vi "random phase generator.vi"(0 "seed":u32=4294967295, 1 "reset":bool) -> (4 "white noise out":i16)   [LabVIEW 2012]
doc: "Generates a white noise signal with uniform or Gaussian distribution.\n--------------------\n\nThis Express VI is configured as follows:\n\n<b>White Noise Type</b>\nUniform\n\n<b>Execution Mode</b>\nOutside single-cycle Timed Loop\n\n<b>Scaling</b>\nAmplitude: 256 \n\n<b>Output Data Type</b>\nI16"
uses:
  <vilib>/Platform/TimedLoop/XDataNode/timing_clust.ctl
  <vilib>/Platform/TimedLoop/XDataNode/nitl_modes.ctl
  <vilib>/Platform/TimedLoop/XDataNode/wakeup.ctl
  <vilib>/rvi/Emulation/niFpgaSctlEmulationRegisterWithScheduler.vi
  <vilib>/rvi/Emulation/niFpgaSctlEmulationScheduler.vi
  <vilib>/Platform/TimedLoop/XDataNode/XDataNode.xnode
  <vilib>/Platform/TimedLoop/XDataNode/XDNodeRunTimeDep.lvlib
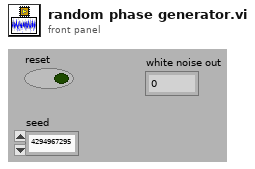
[diagram p1: front panel]
types:
  T1 = typedef "XDNodeRunTimeDep.lvlib/timing_clust.ctl" = cluster{"Expected End [f-1]":u64, "Actual End [f-1]":u64, "Finished Late? [f-1]":bool, "Expected End [i-1]":u64, "Actual End [i-1]":u64, "Finished Late? [i-1]":bool, "Expected Start [i]":u64, "Actual Start [i]":u64, "Expected Start [f]":u64, "Actual Start [f]":u64, "Source Name":string, "Structure Name":string, "Period":i64, "Deadline":i64, "Offset":i64, "Start":i64, "Priority":i32, "Timeout":i32, "Mode":T2, "Wakeup Reason":T3, "Error":errorcluster, "Source Type":string, "Secondary Source Type":string, "Global End Time":u64, "Global Start Time":u64, "Frame Duration":u64, "Iteration Duration":u64, "Assigned CPU":i32, "I/O Scan Engine Mode":u32}
  T2 = typedef "XDNodeRunTimeDep.lvlib/nitl_modes.ctl" = enum32{"No Change", "Process missed periods, maintain original phase", "Discard missed periods, maintain original phase", "Process missed periods, ignore original phase", "Discard missed periods, ignore original phase"}
  T3 = typedef "XDNodeRunTimeDep.lvlib/wakeup.ctl" = enum32{"Normal", "Aborted", "Asynchronous wakeup", "Timing source error", "Timed loop error", "Timeout"}
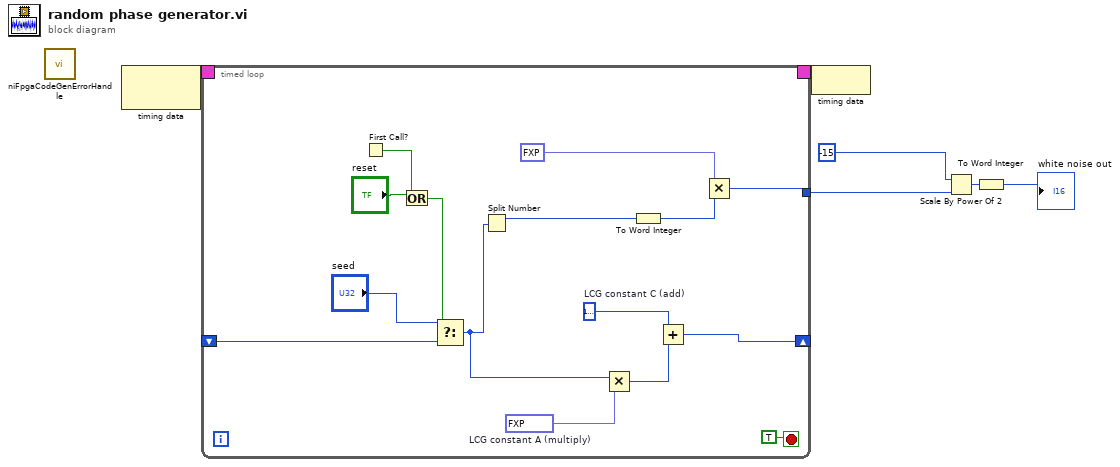
[diagram p0: block diagram]
diagram:
  n1 = call <vilib>:"niFpgaCodeGenErrorHandle.vi"() -> ()  [unwired: 1 in]
  n2 = node-c288() -> (w6:T1)  [unwired: 1 in]
  n3 = timed-loop "Timed Loop" {
    timing: w6 -> [_]
    timing-out: [_] -> w5
    shift-right: [w11] -> _
    shift-left: _ -> [w17]
    tunnel: [w8] -> w3
    stop <- TRUE stop-if-true
    w12 = u32 1013904223  # LCG constant C (add)
    w14 = fxp<+,21,21> 1664525.0  # LCG constant A (multiply)
    n4 = First Call?() -> (First Call?: T/F=w20:bool)
    n5 = Or(x="reset", y=w20) -> (x .or. y?=w18:bool)
    n6 = Select(t="seed", s=w18, f=w17) -> (s? t:f=w16:u32)
    n7 = Split Number(x=w16) -> (hi(x)=w15:u16)  [unwired: 1 out]
    n8 = Multiply(x=w16, y=w14) -> (x*y=w13:u32)
    n9 = To Word Integer(number=w15) -> (16bit integer=w9:i16)
    n10 = Add(x=w13, y=w12) -> (x+y=w11:u32)
    n11 = Multiply(x=fxp<+,9,9> 256.0, y=w9) -> (x*y=w8:i32)
  }
  n12 = node-c288(w5) -> ()
  n13 = Scale By Power Of 2(n=i8 -15 ("Uniform scale factor"), x=w3) -> (x*2^n=w2:i32)
  n14 = To Word Integer(number=w2) -> (16bit integer=→"white noise out":i16)
